vi "synth.vi"() -> ()   [LabVIEW 2025]
uses:
  <vilib>/Waveform/WDTOps.llb/WDT Index Channel DBL.vi
  <vilib>/express/express analysis/Spectral/Block/exnSpectralBlock spectral measurements RMS poly.vi
  <vilib>/express/express analysis/Spectral/Block/exnSpectralBlock spectral measurements RMS DDT.vi
  <vilib>/express/express analysis/Spectral/XNode/ExpressSpectralMeasurementsBlockNode.xnode
panel:
  out "Signal Brut":dynamicdata(graph)
  out "FFT":dynamicdata(graph)
  out "Signal Propre":dynamicdata(graph)
  out "Fréquence":dbl
  out "Note jouée":string
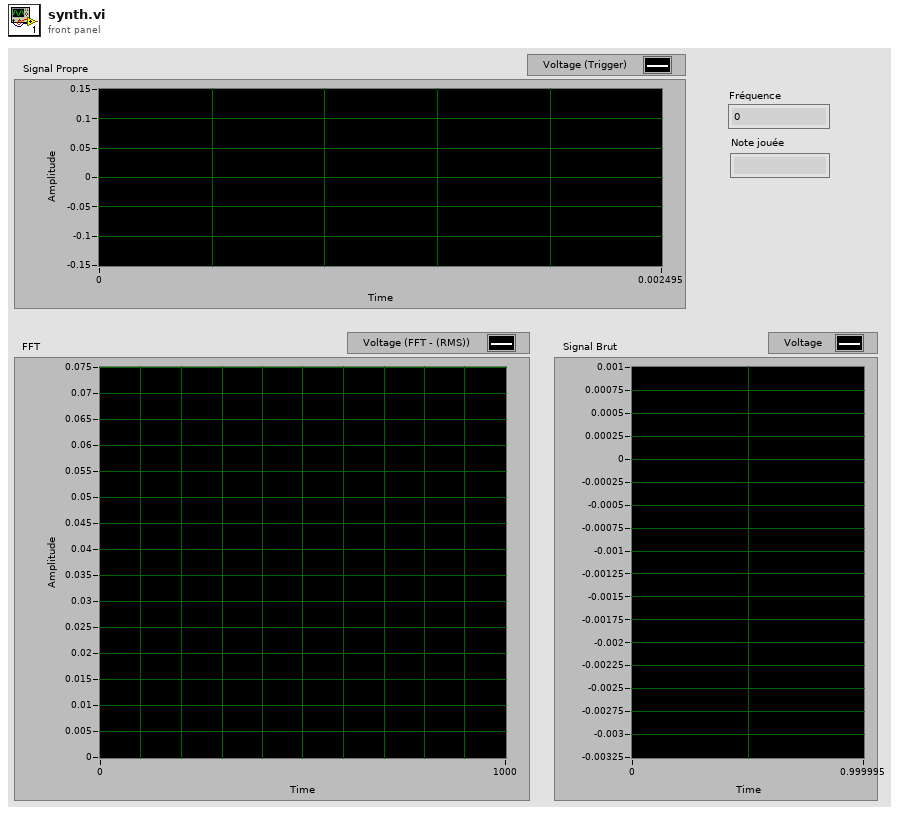
[diagram p1: front panel]
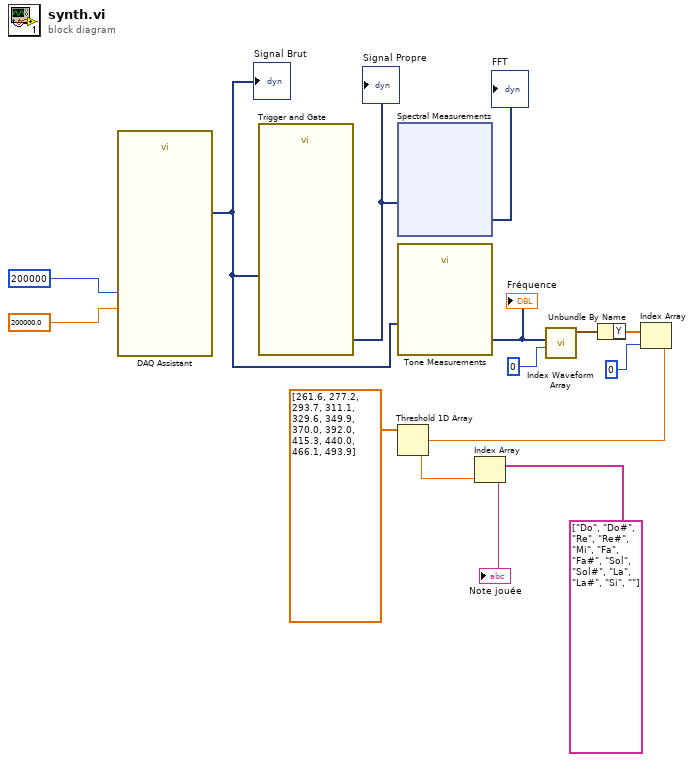
[diagram p0: block diagram]
diagram:
  n1 = call "DAQ Assistant"("rate"=200000.0, "number of samples"=200000) -> ("data"=w2:dynamicdata)  [unwired: 15 in, 2 out]
  "Signal Brut" <- w2
  n2 = call "Trigger and Gate"("Signals"=w2) -> ("Triggered Signals"=w12:dynamicdata)  [unwired: 7 in, 3 out]
  "Signal Propre" <- w12
  n3 = xnode "Spectral Measurements"("Signals"=w12) -> ("FFT - (RMS)"=→"FFT":dynamicdata)  [unwired: 2 in, 3 out]
  n4 = call "Tone Measurements"("Signals"=w2) -> ("Frequency"=w11:dynamicdata)  [unwired: 9 in, 1 out]
  "Fréquence" <- w11
  n5 = call-poly <vilib>:"Index Waveform Array.vi"("index"=0, "waveform array"=w11) -> ("waveform"=w9:waveform(dbl))  [unwired: 8 in, 1 out]
  n6 = Unbundle By Name(w9) -> ("Y"=w8:dbl[])
  n7 = Index Array(array=w8, index=0) -> (element=w5:dbl)
  n8 = Threshold 1D Array(2:w5, 3:dbl[] [261.6, 277.2, 293.7, 311.1, 329.6, 349.9, 370.0, 392.0, 415.3, 440.0, 466.1, 493.9]) -> (0:w3:dbl)  [unwired: 1 in]
  n9 = Index Array(array=string[] ["Do", "Do#", "Re", "Re#", "Mi", "Fa", "Fa#", "Sol", "Sol#", "La", "La#", "Si", ""], index=w3) -> (element=→"Note jouée":string)
